vi "Set String on Multiple Controls.vi"(8 "문자열":string, 11 "Controls":refnum<vi>[](array[refnum]) caption="컨트롤") -> (3 "Controls 2":refnum<vi>[](array[refnum]) caption="컨트롤")   [LabVIEW 2018, in "Library-Ctrl.lvlib"]
uses:
  Library-Ctrl.lvlib
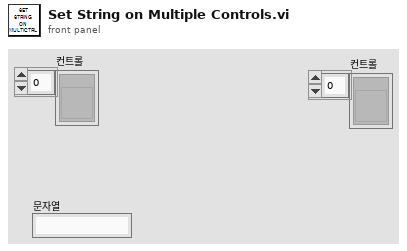
[diagram p1: front panel]
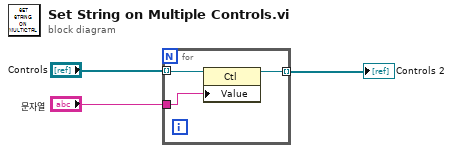
[diagram p0: block diagram]
diagram:
  n1 = for {
    tunnel: "Controls" -> [w6] mode=indexing
    tunnel: [w5] -> w2 mode=indexing
    tunnel: "문자열" -> [w4]
    n2 = property class="Ctl"(reference=w6, "Value"=w4) -> (reference out=w5:refnum<vi>)  [unwired: 1 in, 1 out]
  }
  "Controls 2" <- w2
